vi "Main.vi"(8 "error in (no error)":errorcluster, 11 "TomoBase in":refnum<class "Tomo.lvclass">) -> (0 "error out":errorcluster, 3 "component":refnum<class "Tomo.lvclass">)   [LabVIEW 2012, in "Tomo.lvclass"]
doc: "Main VI of the component."
uses:
  Tomo.lvclass
  <vilib>/Distrio/Murmex/Murmex/command_enum.ctl
  Tomo.lvclass/Tomo.ctl
  <vilib>/Distrio/Murmex/InitialiseMessage/InitialiseMessage.lvclass
  <vilib>/Distrio/Murmex/TerminateMessage/TerminateMessage.lvclass
  <vilib>/Distrio/Murmex/ConfigureMessage/ConfigureMessage.lvclass
  <vilib>/Distrio/Murmex/Murmex/update_cluster.ctl
  <vilib>/Distrio/Murmex/StopMessage/StopMessage.lvclass
  <vilib>/Distrio/Murmex/GenericMessage/GenericMessage.lvclass
  <vilib>/Distrio/Murmex/Murmex/Set configure at initialise.vi
  <vilib>/Distrio/Murmex/Murmex/Set log reference.vi
  <vilib>/Distrio/Murmex/Murmex/Set VI reference.vi
  <vilib>/Distrio/Murmex/Murmex/Set write log to disk.vi
  <vilib>/Distrio/Murmex/Message/Add or replace parameter.vi
  <vilib>/Distrio/Murmex/Murmex/Murmex.lvclass
  <vilib>/Distrio/Murmex/Message/Message.lvclass
panel:
  in  "Tab Control":T1(tab)
  out "TB":dbl format="%#_2g"
  out "Tomography progress":dbl(slide) scale=0.0..1.0
  in  "experiment name":string
  in  "Volume map":T2(ring)
  in  "Z step size":dbl[unit]=1e-06
  in  "X step size":dbl[unit]=0.0005
  in  "Y step size":dbl[unit]=0.0005
  in  "# of views":dbl=1.0
  in  "starting angle":dbl[unit]
  in  "button::start":bool
  out "Estimated remaining time":dbl format="- %<%H:%M:%S>t"
  in  "Default focus":dbl[unit]
  in  "Pivotal X":dbl[unit]
  in  "Reverse stacks?":bool
  in  "X min":dbl[unit]
  in  "X max":dbl[unit]
  in  "Y min":dbl[unit]
  in  "Y max":dbl[unit]
  in  "Z min":dbl[unit]
  in  "Z max":dbl[unit]
  in  "Pre tomo volume file":path
  in  "Pre tomo binary images path":path
  in  "button::pretomo calc":bool
  in  "Custom volume path":path
  in  "Experimenter email address":string
  in  "Experimenter name":string
  in  "generic command":string
  in  "button::send command":bool
  out "log":string
  in  "ID":string="tomo"
  in  "command":T3
  in  "recipient":string
  in  "button::configure":bool
  in  "button::quit":bool
  in  "terminate?":bool
  # "Tomo\n\nImplemented by:\nLudovico Silvestri\nUniversity of Florence, Italy"
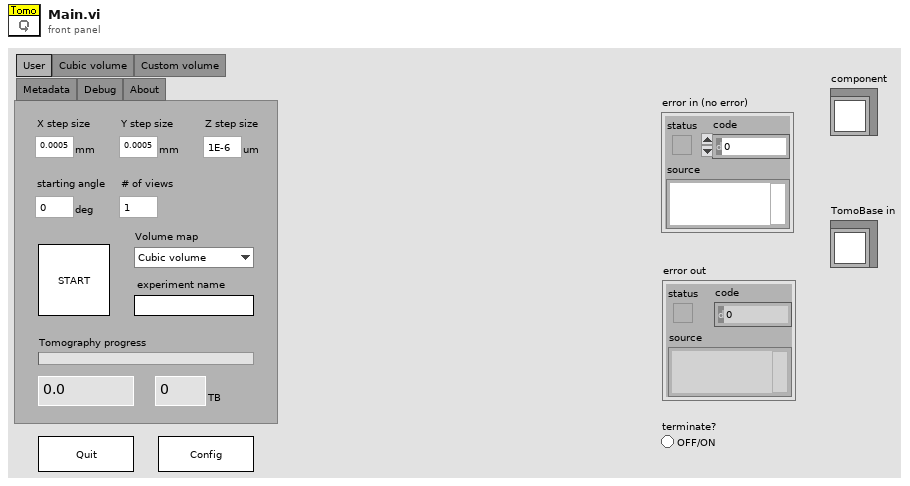
[diagram p1: front panel]
types:
  T1 = enum32{"User", "Cubic volume", "Custom volume", "Metadata", "Debug", "About"}
  T2 = enum16{"Cubic volume", "Custom volume", "Self-generate volume"}
  T3 = typedef "Murmex.lvlib/Murmex.lvclass/command_enum.ctl" = enum16{"null", "initialise", "reset", "terminate", "acknowledge", "update", "inspect", "inform", "proceed", "start", "stop", "fetch", "configure", "generic"}
  T4 = typedef "Murmex.lvlib/Murmex.lvclass/update_cluster.ctl" = cluster{"target ID":string, "key chains":string[], "values":variant[]}
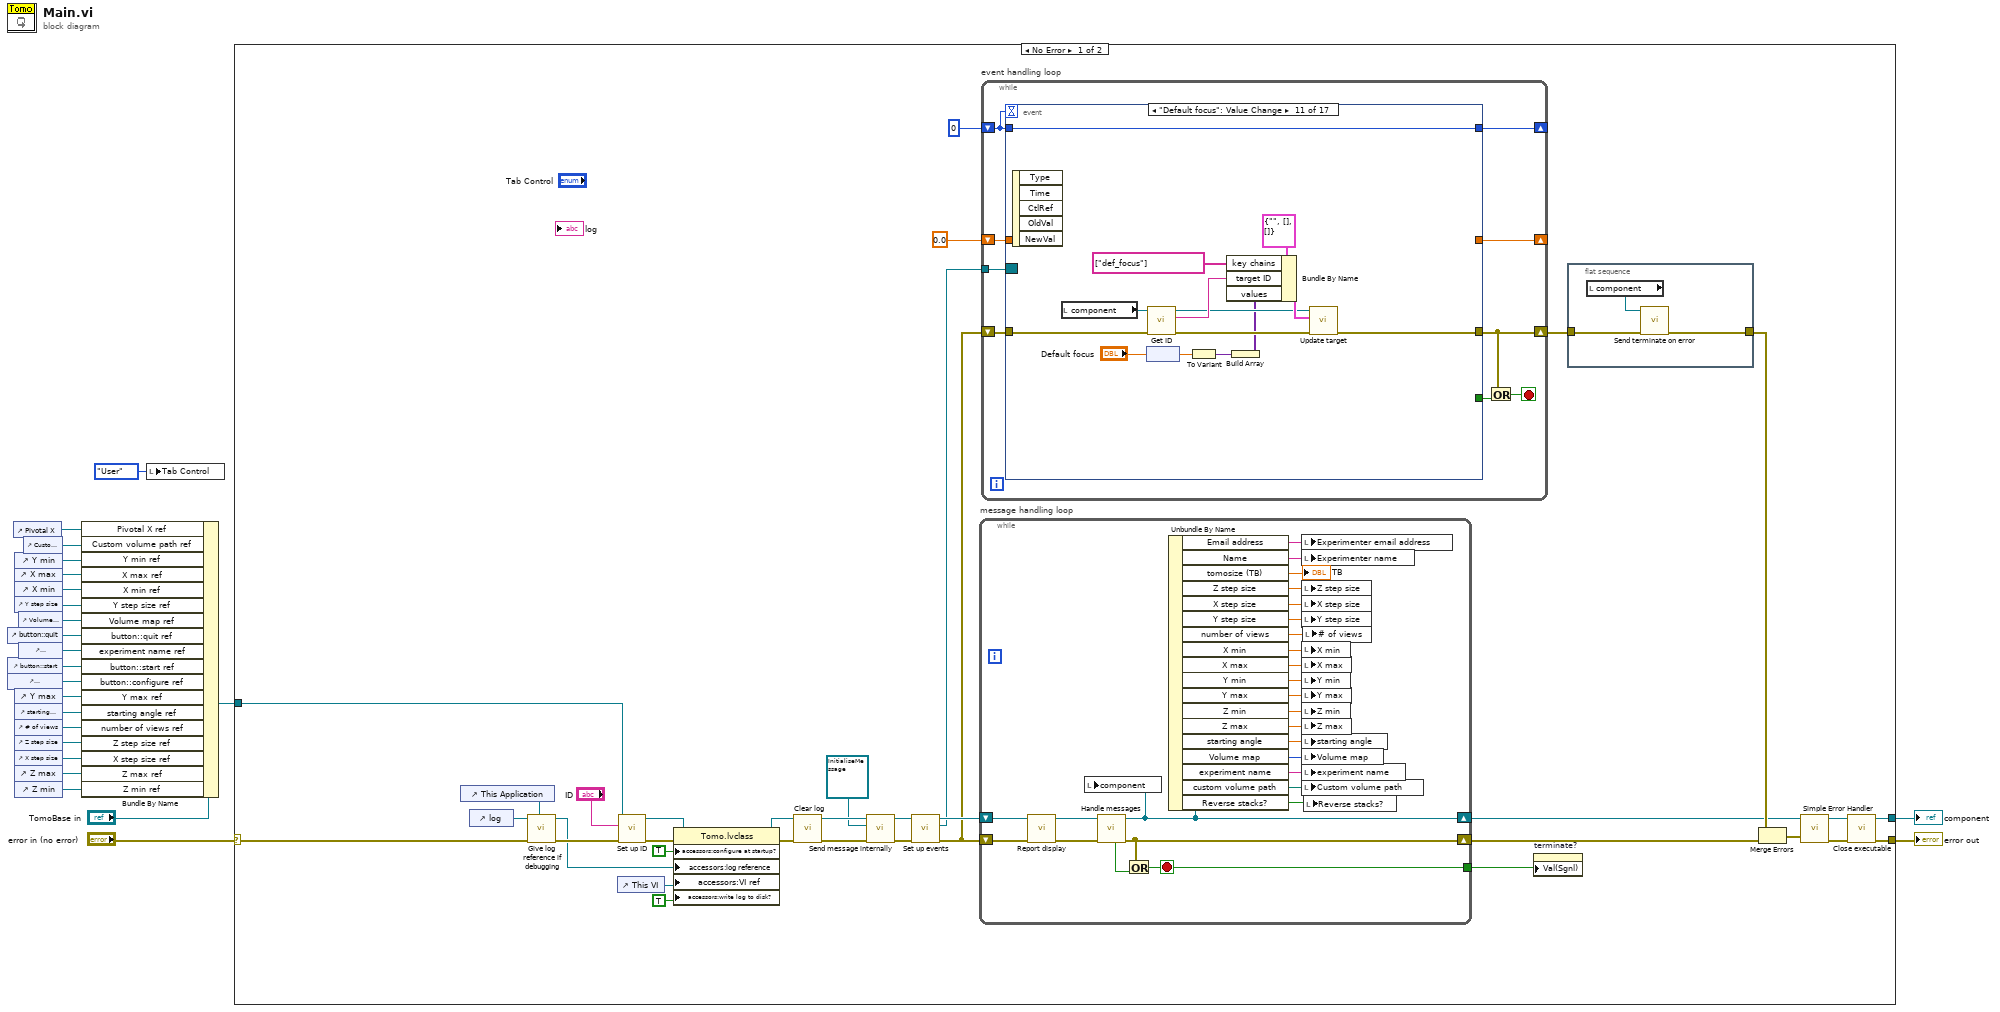
[diagram p0: block diagram]
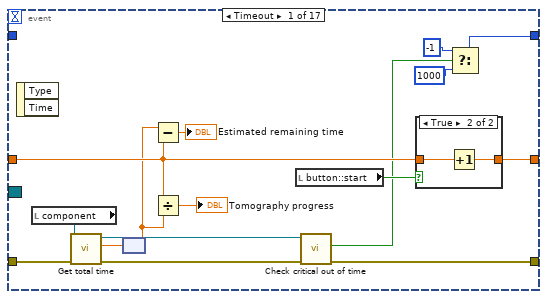
[diagram p2: hidden frame]
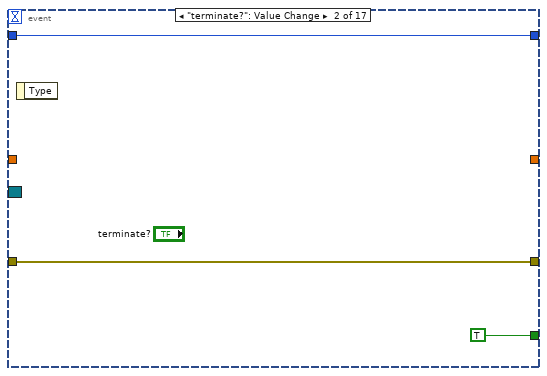
[diagram p4: hidden frame]
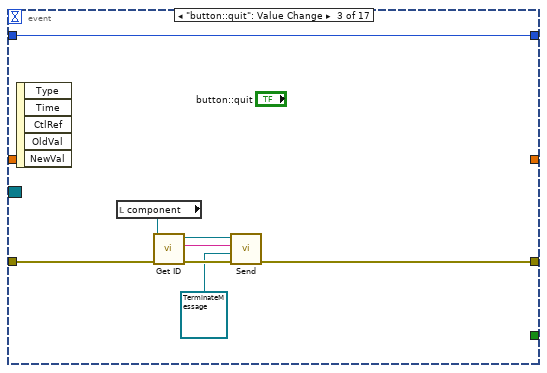
[diagram p5: hidden frame]
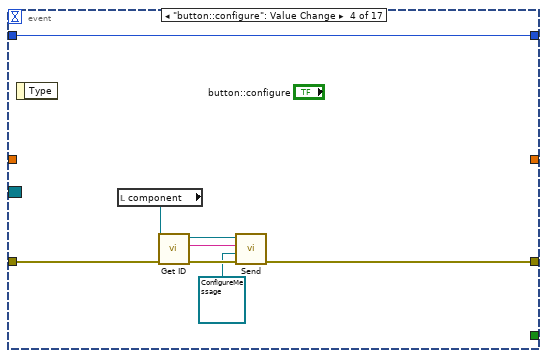
[diagram p6: hidden frame]
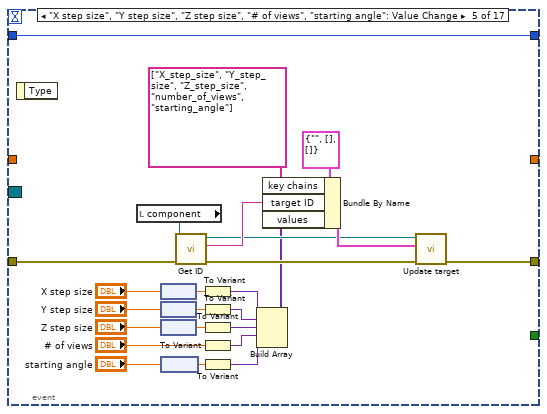
[diagram p7: hidden frame]
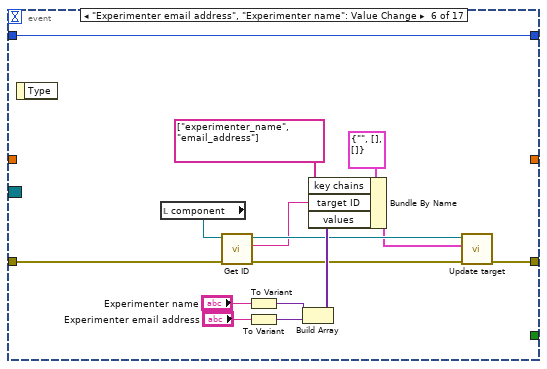
[diagram p8: hidden frame]
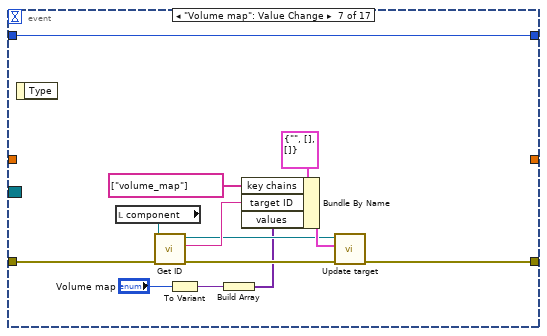
[diagram p9: hidden frame]
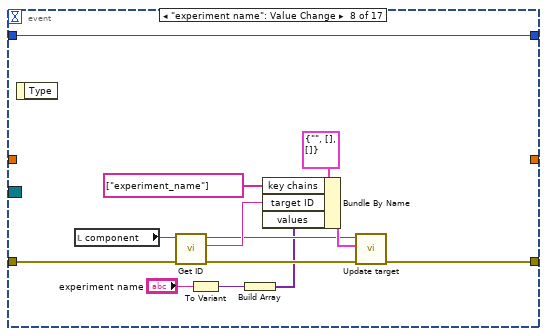
[diagram p10: hidden frame]
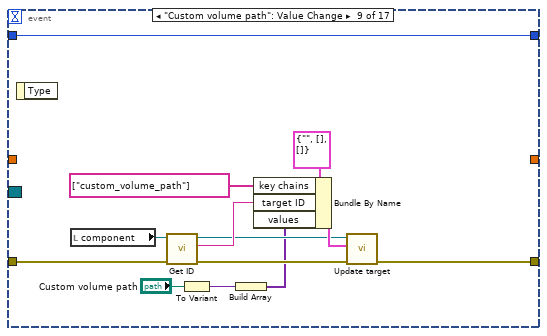
[diagram p11: hidden frame]
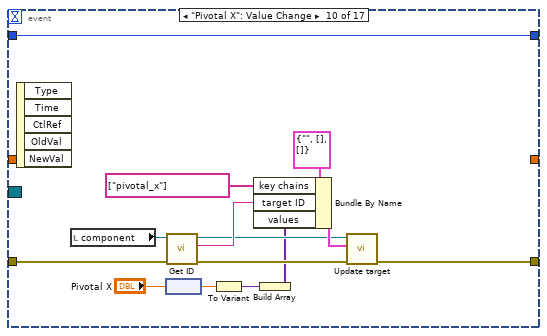
[diagram p12: hidden frame]
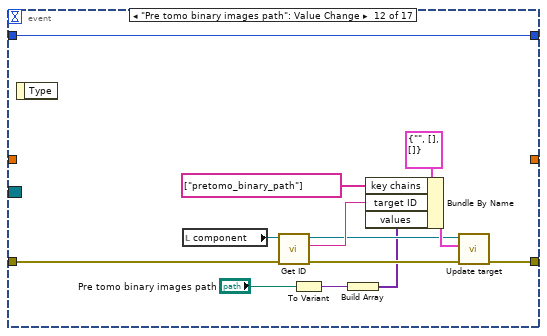
[diagram p13: hidden frame]
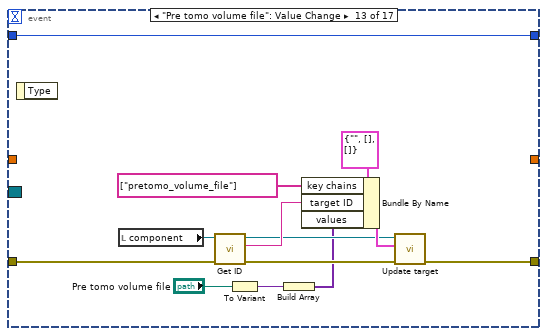
[diagram p14: hidden frame]
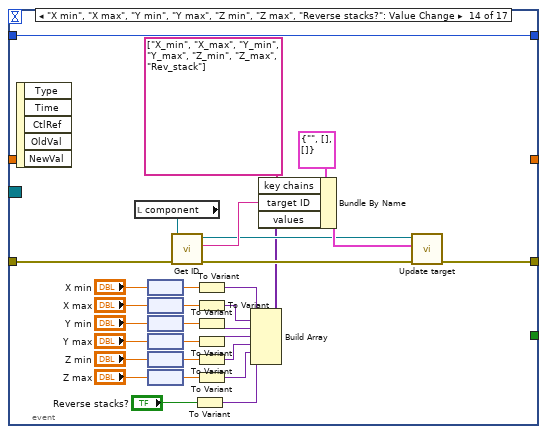
[diagram p15: hidden frame]
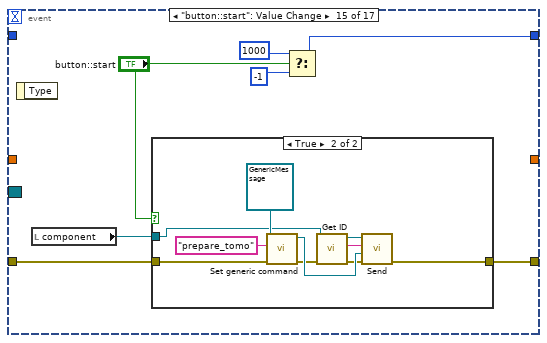
[diagram p16: hidden frame]
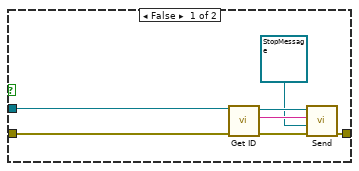
[diagram p17: hidden frame]
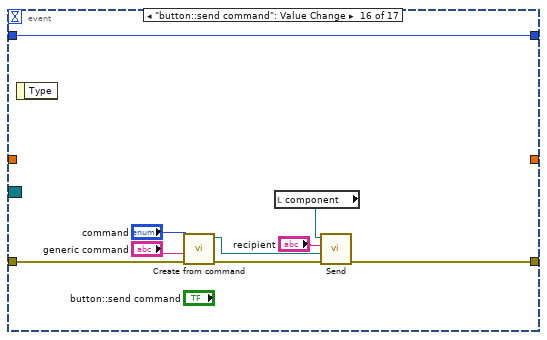
[diagram p18: hidden frame]
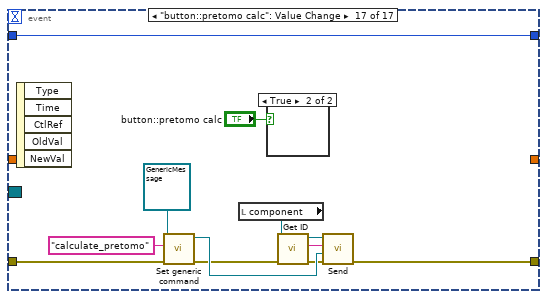
[diagram p19: hidden frame]
diagram:
  n1 = control-ref of="button::quit"() -> (w13:refnum<vi>)
  n2 = control-ref of="button::start"() -> (w11:refnum<vi>)
  n3 = control-ref of="button::configure"() -> (w10:refnum<vi>)
  n4 = control-ref of="Pivotal X"() -> (w1:refnum<vi>)
  n5 = control-ref of="Y min"() -> (w18:refnum<vi>)
  n6 = control-ref of="X max"() -> (w17:refnum<vi>)
  n7 = control-ref of="X min"() -> (w16:refnum<vi>)
  n8 = control-ref of="Y step size"() -> (w15:refnum<vi>)
  n9 = control-ref of="Y max"() -> (w9:refnum<vi>)
  n10 = control-ref of="starting angle"() -> (w8:refnum<vi>)
  n11 = control-ref of="# of views"() -> (w7:refnum<vi>)
  n12 = control-ref of="Z step size"() -> (w6:refnum<vi>)
  n13 = control-ref of="X step size"() -> (w5:refnum<vi>)
  n14 = control-ref of="Z max"() -> (w4:refnum<vi>)
  n15 = control-ref of="Z min"() -> (w3:refnum<vi>)
  n16 = control-ref of="Volume map"() -> (w14:refnum<vi>)
  n17 = control-ref of="experiment name"() -> (w12:refnum<vi>)
  n18 = control-ref of="Custom volume path"() -> (w19:refnum<vi>)
  n19 = Bundle By Name(cluster="TomoBase in", "Pivotal X ref"=w1, "Custom volume path ref"=w19, "Y min ref"=w18, "X max ref"=w17, "X min ref"=w16, "Y step size ref"=w15, "Volume map ref"=w14, "button::quit ref"=w13, "experiment name ref"=w12, "button::start ref"=w11, "button::configure ref"=w10, "Y max ref"=w9, "starting angle ref"=w8, "number of views ref"=w7, "Z step size ref"=w6, "X step size ref"=w5, "Z max ref"=w4, "Z min ref"=w3) -> (w20:refnum<class "Tomo.lvclass">)
  n20 = local write "Tab Control"(T1."User" ("Tab Control")) -> ()
  n21 = case shown="No Error" "error in (no error)" {
    selector: "error in (no error)" -> [w29 w343]
    tunnel: w20 -> [w54 w342]
    tunnel: [w34 w343] -> w23
    tunnel: [w32 w342] -> w22
    frame No Error {
      n22 = control-ref of="This Application"() -> (w26:refnum<vi>)
      n23 = control-ref of="log"() -> (w28:refnum<vi>)
      n24 = call "Give log reference if debugging.vi"("application ref"=w26, "error in (no error)"=w29, "log reference in"=w28) -> ("error out"=w30:errorcluster, "log reference out"=w27:refnum<vi>)  [unwired: 6 in, 1 out]
      n25 = control-ref of="This VI"() -> (w56:refnum<vi>)
      n26 = call <vilib>:"Set up ID.vi"("error in (no error)"=w30, "component ID"="ID", "MurmexBase in"=w54) -> ("error out"=w55:errorcluster, "MurmexBase out"=w52:refnum<class "Tomo.lvclass">)  [unwired: 6 in, 1 out]
      n27 = property class="Tomo.lvclass"(reference=w52, error in=w55, "accessors:configure at startup?"=TRUE ("configure at startup?"), "accessors:log reference"=w27, "accessors:VI ref"=w56, "accessors:write log to disk?"=TRUE ("write log to disk?")) -> (reference out=w50:refnum<class "Tomo.lvclass">, error out=w51:errorcluster)
      n28 = call <vilib>:"Clear log.vi"("error in (no error)"=w51, "MurmexBase in"=w50) -> ("error out"=w49:errorcluster, "MurmexBase out"=w48:refnum<class "Tomo.lvclass">)  [unwired: 8 in]
      n29 = call <vilib>:"Send message internally.vi"("error in (no error)"=w49, "Message"=refnum<class "InitialiseMessage.lvclass"> refnum ("Message in"), "Murmex in"=w48) -> ("error out"=w46:errorcluster, "Murmex out"=w45:refnum<class "Tomo.lvclass">)  [unwired: 7 in]
      n30 = call <vilib>:"Set up events.vi"("error in (no error)"=w46, "MurmexBase in"=w45) -> ("error out"=w43:errorcluster, "Event Registration Refnum"=w42:refnum<event-registration>, "MurmexBase out"=w44:refnum<class "Tomo.lvclass">)  [unwired: 7 in]
      n31 = while "message handling loop" {
        shift-right: [w322] -> w39
        shift-left: w43 -> [w320]
        shift-right: [w321] -> w33
        shift-left: w44 -> [w318]
        tunnel: [w340] -> w35
        stop <- w340 stop-if-true
        n32 = call-dynamic "Report display.vi"("error in (no error)"=w320, "Tomo in"=w318) -> ("error out"=w319:errorcluster, "Tomo out"=w317:refnum<class "Tomo.lvclass">)  [unwired: 8 in]
        n33 = call <vilib>:"Handle messages.vi"("error in (no error)"=w319, "Murmex in"=w317) -> ("error out"=w322:errorcluster, "Murmex out"=w321:refnum<class "Tomo.lvclass">, "terminated?"=w341:bool)  [unwired: 7 in]
        n34 = local write "component"(w321) -> ()
        n35 = Or(x=w322, y=w341) -> (x .or. y?=w340:bool)
        n36 = Unbundle By Name(w321) -> ("Email address"=w323:string, "Name"=w324:string, "tomosize (TB)"=→"TB":dbl, "Z step size"=w331:dbl[unit], "X step size"=w333:dbl[unit], "Y step size"=w332:dbl[unit], "number of views"=w330:dbl, "X min"=w339:dbl[unit], "X max"=w338:dbl[unit], "Y min"=w337:dbl[unit], "Y max"=w336:dbl[unit], "Z min"=w335:dbl[unit], "Z max"=w334:dbl[unit], "starting angle"=w329:dbl[unit], "Volume map"=w328:T2, "experiment name"=w327:string, "custom volume path"=w326:path, "Reverse stacks?"=w316:bool)
        n37 = local write "Experimenter email address"(w323) -> ()
        n38 = local write "Experimenter name"(w324) -> ()
        n39 = local write "Z step size"(w331) -> ()
        n40 = local write "X step size"(w333) -> ()
        n41 = local write "Y step size"(w332) -> ()
        n42 = local write "X min"(w339) -> ()
        n43 = local write "X max"(w338) -> ()
        n44 = local write "Y min"(w337) -> ()
        n45 = local write "Y max"(w336) -> ()
        n46 = local write "Z min"(w335) -> ()
        n47 = local write "Z max"(w334) -> ()
        n48 = local write "starting angle"(w329) -> ()
        n49 = local write "Volume map"(w328) -> ()
        n50 = local write "experiment name"(w327) -> ()
        n51 = local write "Custom volume path"(w326) -> ()
        n52 = local write "# of views"(w330) -> ()
        n53 = local write "Reverse stacks?"(w316) -> ()
      }
      n54 = while "event handling loop" {
        shift-right: [w64] -> w40
        shift-left: w43 -> [w69]
        tunnel: w42 -> [w68]
        shift-right: [w66] -> _
        shift-left: 0 -> [w67]
        shift-right: [w61] -> _
        shift-left: 0.0 -> [w62]
        stop <- w63 stop-if-true
        n55 = event shown="[10] \"Default focus\": Value Change" {
          selector: w68 -> [_ _ _ _ _ _ _ _ _ _ _ _ _ _ _ _ _]
          dyn-events: _ -> [_ _ _ _ _ _ _ _ _ _ _ _ _ _ _ _ _]
          timeout: w67 -> [_ _ _ _ _ _ _ _ _ _ _ _ _ _ _ _ _]
          tunnel: [w75 w89 w96 w102 w130 w138 w154 w162 w178 w192 w206 w219 w232 w265 w277 w296 w306] -> w64
          tunnel: w69 -> [w85 w89 w98 w103 w128 w137 w156 w165 w177 w191 w205 w218 w231 w263 w276 w302 w307]
          tunnel: w67 -> [_ w88 w91 w99 w111 w132 w153 w161 w173 w188 w202 w215 w228 w249 _ w295 w304]
          tunnel: [w70 w88 w91 w99 w111 w132 w153 w161 w173 w188 w202 w215 w228 w249 w271 w295 w304] -> w66
          tunnel: [_ TRUE _ _ _ _ _ _ _ _ _ _ _ _ _ _ _] -> w65
          tunnel: w62 -> [w83 _ _ _ _ _ _ _ _ _ _ _ _ _ _ _ _]
          tunnel: [w82 _ _ _ _ _ _ _ _ _ _ _ _ _ _ _ _] -> w61
          event Timeout {
            n56 = event-data() -> ()  [unwired: 1 in, 2 out]
            n57 = local read "component"() -> (w81:refnum<class "Tomo.lvclass">)
            n58 = call-dynamic "Get total time.vi"("error in (no error)"=w85, "Tomo in"=w81) -> ("error out"=w84:errorcluster, "Total time"=w80:dbl[unit], "Tomo out"=w74:refnum<class "Tomo.lvclass">)  [unwired: 7 in]
            n59 = node(w80) -> (w78:dbl)
            n60 = Subtract(x=w78, y=w83) -> (x-y=→"Estimated remaining time":dbl)
            n61 = Divide(x=w83, y=w78) -> (x/y=→"Tomography progress":dbl)
            n62 = local read "button::start"() -> (w76:bool)
            n63 = call-dynamic "Check critical out of time.vi"("error in (no error)"=w84, "Tomo in"=w74) -> ("error out"=w75:errorcluster, "critical issue?"=w73:bool)  [unwired: 7 in, 1 out]
            n64 = case shown="True" w76 {
              tunnel: w83 -> [_ w87]
              tunnel: [_ w86] -> w82
              frame False {
              }
              frame True {
                n65 = Increment(x=w87) -> (x+1=w86:dbl)
              }
            }
            n66 = Select(t=-1, s=w73, f=1000) -> (s? t:f=w70:i32)
          }
          event "terminate?": Value Change {
            n67 = event-data() -> ()  [unwired: 1 in, 1 out]
          }
          event "button::quit": Value Change {
            n68 = event-data() -> ()  [unwired: 1 in, 5 out]
            n69 = local read "component"() -> (w95:refnum<class "Tomo.lvclass">)
            n70 = call <vilib>:"Get ID.vi"("error in (no error)"=w98, "Murmex in"=w95) -> ("error out"=w97:errorcluster, "component id"=w93:string, "Murmex out"=w94:refnum<class "Tomo.lvclass">)  [unwired: 7 in]
            n71 = call <vilib>:"Send.vi"("error in (no error)"=w97, "Message"=refnum<class "TerminateMessage.lvclass"> refnum ("Distrio Murmex 1.1:TerminateMessage"), "recipient"=w93, "Murmex in"=w94) -> ("error out"=w96:errorcluster)  [unwired: 6 in, 1 out]
          }
          event "button::configure": Value Change {
            n72 = event-data() -> ()  [unwired: 1 in, 1 out]
            n73 = local read "component"() -> (w101:refnum<class "Tomo.lvclass">)
            n74 = call <vilib>:"Get ID.vi"("error in (no error)"=w103, "Murmex in"=w101) -> ("error out"=w106:errorcluster, "component id"=w104:string, "Murmex out"=w105:refnum<class "Tomo.lvclass">)  [unwired: 7 in]
            n75 = call <vilib>:"Send.vi"("error in (no error)"=w106, "Message"=refnum<class "ConfigureMessage.lvclass"> refnum ("Distrio Murmex 1.1:ConfigureMessage"), "recipient"=w104, "Murmex in"=w105) -> ("error out"=w102:errorcluster)  [unwired: 6 in, 1 out]
          }
          event "X step size", "Y step size", "Z step size", "# of views", "starting angle": Value Change {
            n76 = event-data() -> ()  [unwired: 1 in, 1 out]
            n77 = local read "component"() -> (w126:refnum<class "Tomo.lvclass">)
            n78 = node("X step size") -> (w110:dbl)
            n79 = node("Y step size") -> (w109:dbl)
            n80 = node("Z step size") -> (w108:dbl)
            n81 = node("starting angle") -> (w107:dbl)
            n82 = call <vilib>:"Get ID.vi"("error in (no error)"=w128, "Murmex in"=w126) -> ("error out"=w129:errorcluster, "component id"=w127:string, "Murmex out"=w124:refnum<class "Tomo.lvclass">)  [unwired: 7 in]
            n83 = To Variant(anything=w110) -> (Variant=w114:variant)
            n84 = To Variant(anything=w109) -> (Variant=w115:variant)
            n85 = To Variant(anything=w108) -> (Variant=w118:variant)
            n86 = To Variant(anything="# of views") -> (Variant=w117:variant)
            n87 = To Variant(anything=w107) -> (Variant=w116:variant)
            n88 = Build Array(w114, w115, w118, w117, w116) -> (w113:variant[])
            n89 = Bundle By Name(cluster=T4 {"target ID"="", "key chains"=[], "values"=[]} ("update cluster"), "key chains"=string[] ["X_step_size", "Y_step_size", "Z_step_size", "number_of_views", "starting_angle"], "target ID"=w127, "values"=w113) -> (w125:T4)
            n90 = call <vilib>:"Update target.vi"("error in (no error)"=w129, "update cluster"=w125, "MurmexBase in"=w124) -> ("error out"=w130:errorcluster)  [unwired: 7 in, 1 out]
          }
          event "Experimenter email address", "Experimenter name": Value Change {
            n91 = event-data() -> ()  [unwired: 1 in, 1 out]
            n92 = local read "component"() -> (w133:refnum<class "Tomo.lvclass">)
            n93 = call <vilib>:"Get ID.vi"("error in (no error)"=w137, "Murmex in"=w133) -> ("error out"=w140:errorcluster, "component id"=w141:string, "Murmex out"=w143:refnum<class "Tomo.lvclass">)  [unwired: 7 in]
            n94 = To Variant(anything="Experimenter name") -> (Variant=w145:variant)
            n95 = To Variant(anything="Experimenter email address") -> (Variant=w144:variant)
            n96 = Build Array(w145, w144) -> (w146:variant[])
            n97 = Bundle By Name(cluster=T4 {"target ID"="", "key chains"=[], "values"=[]} ("update cluster"), "key chains"=string[] ["experimenter_name", "email_address"], "target ID"=w141, "values"=w146) -> (w142:T4)
            n98 = call <vilib>:"Update target.vi"("error in (no error)"=w140, "update cluster"=w142, "MurmexBase in"=w143) -> ("error out"=w138:errorcluster)  [unwired: 7 in, 1 out]
          }
          event "Volume map": Value Change {
            n99 = event-data() -> ()  [unwired: 1 in, 1 out]
            n100 = local read "component"() -> (w147:refnum<class "Tomo.lvclass">)
            n101 = call <vilib>:"Get ID.vi"("error in (no error)"=w156, "Murmex in"=w147) -> ("error out"=w155:errorcluster, "component id"=w159:string, "Murmex out"=w157:refnum<class "Tomo.lvclass">)  [unwired: 7 in]
            n102 = To Variant(anything="Volume map") -> (Variant=w152:variant)
            n103 = Build Array(w152) -> (w151:variant[])
            n104 = Bundle By Name(cluster=T4 {"target ID"="", "key chains"=[], "values"=[]} ("update cluster"), "key chains"=string[] ["volume_map"], "target ID"=w159, "values"=w151) -> (w158:T4)
            n105 = call <vilib>:"Update target.vi"("error in (no error)"=w155, "update cluster"=w158, "MurmexBase in"=w157) -> ("error out"=w154:errorcluster)  [unwired: 7 in, 1 out]
          }
          event "experiment name": Value Change {
            n106 = event-data() -> ()  [unwired: 1 in, 1 out]
            n107 = local read "component"() -> (w160:refnum<class "Tomo.lvclass">)
            n108 = call <vilib>:"Get ID.vi"("error in (no error)"=w165, "Murmex in"=w160) -> ("error out"=w169:errorcluster, "component id"=w172:string, "Murmex out"=w170:refnum<class "Tomo.lvclass">)  [unwired: 7 in]
            n109 = To Variant(anything="experiment name") -> (Variant=w168:variant)
            n110 = Build Array(w168) -> (w167:variant[])
            n111 = Bundle By Name(cluster=T4 {"target ID"="", "key chains"=[], "values"=[]} ("update cluster"), "key chains"=string[] ["experiment_name"], "target ID"=w172, "values"=w167) -> (w171:T4)
            n112 = call <vilib>:"Update target.vi"("error in (no error)"=w169, "update cluster"=w171, "MurmexBase in"=w170) -> ("error out"=w162:errorcluster)  [unwired: 7 in, 1 out]
          }
          event "Custom volume path": Value Change {
            n113 = event-data() -> ()  [unwired: 1 in, 1 out]
            n114 = local read "component"() -> (w175:refnum<class "Tomo.lvclass">)
            n115 = call <vilib>:"Get ID.vi"("error in (no error)"=w177, "Murmex in"=w175) -> ("error out"=w182:errorcluster, "component id"=w185:string, "Murmex out"=w183:refnum<class "Tomo.lvclass">)  [unwired: 7 in]
            n116 = To Variant(anything="Custom volume path") -> (Variant=w181:variant)
            n117 = Build Array(w181) -> (w180:variant[])
            n118 = Bundle By Name(cluster=T4 {"target ID"="", "key chains"=[], "values"=[]} ("update cluster"), "key chains"=string[] ["custom_volume_path"], "target ID"=w185, "values"=w180) -> (w184:T4)
            n119 = call <vilib>:"Update target.vi"("error in (no error)"=w182, "update cluster"=w184, "MurmexBase in"=w183) -> ("error out"=w178:errorcluster)  [unwired: 7 in, 1 out]
          }
          event "Pivotal X": Value Change {
            n120 = event-data() -> ()  [unwired: 1 in, 5 out]
            n121 = local read "component"() -> (w190:refnum<class "Tomo.lvclass">)
            n122 = node("Pivotal X") -> (w186:dbl)
            n123 = call <vilib>:"Get ID.vi"("error in (no error)"=w191, "Murmex in"=w190) -> ("error out"=w196:errorcluster, "component id"=w199:string, "Murmex out"=w197:refnum<class "Tomo.lvclass">)  [unwired: 7 in]
            n124 = To Variant(anything=w186) -> (Variant=w195:variant)
            n125 = Build Array(w195) -> (w194:variant[])
            n126 = Bundle By Name(cluster=T4 {"target ID"="", "key chains"=[], "values"=[]} ("update cluster"), "key chains"=string[] ["pivotal_x"], "target ID"=w199, "values"=w194) -> (w198:T4)
            n127 = call <vilib>:"Update target.vi"("error in (no error)"=w196, "update cluster"=w198, "MurmexBase in"=w197) -> ("error out"=w192:errorcluster)  [unwired: 7 in, 1 out]
          }
          event "Default focus": Value Change {
            n128 = event-data() -> ()  [unwired: 1 in, 5 out]
            n129 = local read "component"() -> (w204:refnum<class "Tomo.lvclass">)
            n130 = node("Default focus") -> (w201:dbl)
            n131 = call <vilib>:"Get ID.vi"("error in (no error)"=w205, "Murmex in"=w204) -> ("error out"=w210:errorcluster, "component id"=w213:string, "Murmex out"=w211:refnum<class "Tomo.lvclass">)  [unwired: 7 in]
            n132 = To Variant(anything=w201) -> (Variant=w209:variant)
            n133 = Build Array(w209) -> (w208:variant[])
            n134 = Bundle By Name(cluster=T4 {"target ID"="", "key chains"=[], "values"=[]} ("update cluster"), "key chains"=string[] ["def_focus"], "target ID"=w213, "values"=w208) -> (w212:T4)
            n135 = call <vilib>:"Update target.vi"("error in (no error)"=w210, "update cluster"=w212, "MurmexBase in"=w211) -> ("error out"=w206:errorcluster)  [unwired: 7 in, 1 out]
          }
          event "Pre tomo binary images path": Value Change {
            n136 = event-data() -> ()  [unwired: 1 in, 1 out]
            n137 = local read "component"() -> (w217:refnum<class "Tomo.lvclass">)
            n138 = call <vilib>:"Get ID.vi"("error in (no error)"=w218, "Murmex in"=w217) -> ("error out"=w223:errorcluster, "component id"=w226:string, "Murmex out"=w224:refnum<class "Tomo.lvclass">)  [unwired: 7 in]
            n139 = To Variant(anything="Pre tomo binary images path") -> (Variant=w222:variant)
            n140 = Build Array(w222) -> (w221:variant[])
            n141 = Bundle By Name(cluster=T4 {"target ID"="", "key chains"=[], "values"=[]} ("update cluster"), "key chains"=string[] ["pretomo_binary_path"], "target ID"=w226, "values"=w221) -> (w225:T4)
            n142 = call <vilib>:"Update target.vi"("error in (no error)"=w223, "update cluster"=w225, "MurmexBase in"=w224) -> ("error out"=w219:errorcluster)  [unwired: 7 in, 1 out]
          }
          event "Pre tomo volume file": Value Change {
            n143 = event-data() -> ()  [unwired: 1 in, 1 out]
            n144 = local read "component"() -> (w230:refnum<class "Tomo.lvclass">)
            n145 = call <vilib>:"Get ID.vi"("error in (no error)"=w231, "Murmex in"=w230) -> ("error out"=w236:errorcluster, "component id"=w239:string, "Murmex out"=w237:refnum<class "Tomo.lvclass">)  [unwired: 7 in]
            n146 = To Variant(anything="Pre tomo volume file") -> (Variant=w235:variant)
            n147 = Build Array(w235) -> (w234:variant[])
            n148 = Bundle By Name(cluster=T4 {"target ID"="", "key chains"=[], "values"=[]} ("update cluster"), "key chains"=string[] ["pretomo_volume_file"], "target ID"=w239, "values"=w234) -> (w238:T4)
            n149 = call <vilib>:"Update target.vi"("error in (no error)"=w236, "update cluster"=w238, "MurmexBase in"=w237) -> ("error out"=w232:errorcluster)  [unwired: 7 in, 1 out]
          }
          event "X min", "X max", "Y min", "Y max", "Z min", "Z max", "Reverse stacks?": Value Change {
            n150 = event-data() -> ()  [unwired: 1 in, 5 out]
            n151 = local read "component"() -> (w262:refnum<class "Tomo.lvclass">)
            n152 = node("X min") -> (w248:dbl)
            n153 = node("X max") -> (w247:dbl)
            n154 = node("Y min") -> (w246:dbl)
            n155 = node("Y max") -> (w245:dbl)
            n156 = node("Z min") -> (w243:dbl)
            n157 = node("Z max") -> (w242:dbl)
            n158 = call <vilib>:"Get ID.vi"("error in (no error)"=w263, "Murmex in"=w262) -> ("error out"=w264:errorcluster, "component id"=w269:string, "Murmex out"=w267:refnum<class "Tomo.lvclass">)  [unwired: 7 in]
            n159 = To Variant(anything="Reverse stacks?") -> (Variant=w240:variant)
            n160 = To Variant(anything=w248) -> (Variant=w258:variant)
            n161 = To Variant(anything=w247) -> (Variant=w259:variant)
            n162 = To Variant(anything=w246) -> (Variant=w261:variant)
            n163 = To Variant(anything=w245) -> (Variant=w260:variant)
            n164 = To Variant(anything=w243) -> (Variant=w251:variant)
            n165 = To Variant(anything=w242) -> (Variant=w250:variant)
            n166 = Build Array(w258, w259, w261, w260, w251, w250, w240) -> (w257:variant[])
            n167 = Bundle By Name(cluster=T4 {"target ID"="", "key chains"=[], "values"=[]} ("update cluster"), "key chains"=string[] ["X_min", "X_max", "Y_min", "Y_max", "Z_min", "Z_max", "Rev_stack"], "target ID"=w269, "values"=w257) -> (w268:T4)
            n168 = call <vilib>:"Update target.vi"("error in (no error)"=w264, "update cluster"=w268, "MurmexBase in"=w267) -> ("error out"=w265:errorcluster)  [unwired: 7 in, 1 out]
          }
          event "button::start": Value Change {
            n169 = event-data() -> ()  [unwired: 1 in, 1 out]
            n170 = local read "component"() -> (w275:refnum<class "Tomo.lvclass">)
            n171 = case shown="True" "button::start" {
              tunnel: [w282 w285] -> w277
              tunnel: w276 -> [w280 w287]
              tunnel: w275 -> [w278 w286]
              frame False {
                n172 = call <vilib>:"Get ID.vi"("error in (no error)"=w280, "Murmex in"=w278) -> ("error out"=w281:errorcluster, "component id"=w283:string, "Murmex out"=w284:refnum<class "Tomo.lvclass">)  [unwired: 7 in]
                n173 = call <vilib>:"Send.vi"("error in (no error)"=w281, "Message"=refnum<class "StopMessage.lvclass"> refnum ("Distrio Murmex 1.1:StopMessage"), "recipient"=w283, "Murmex in"=w284) -> ("error out"=w282:errorcluster)  [unwired: 6 in, 1 out]
              }
              frame True {
                n174 = call <vilib>:"Set generic command.vi"("error in (no error)"=w287, "generic command"="prepare_tomo", "GenericMessage in"=refnum<class "GenericMessage.lvclass"> refnum ("Message in")) -> ("error out"=w289:errorcluster, "GenericMessage out"=w293:refnum<class "GenericMessage.lvclass">)  [unwired: 7 in]
                n175 = call <vilib>:"Get ID.vi"("error in (no error)"=w289, "Murmex in"=w286) -> ("error out"=w290:errorcluster, "component id"=w292:string, "Murmex out"=w291:refnum<class "Tomo.lvclass">)  [unwired: 7 in]
                n176 = call <vilib>:"Send.vi"("error in (no error)"=w290, "Message"=w293, "recipient"=w292, "Murmex in"=w291) -> ("error out"=w285:errorcluster)  [unwired: 6 in, 1 out]
              }
            }
            n177 = Select(t=1000, s="button::start", f=-1) -> (s? t:f=w271:i32)
          }
          event "button::send command": Value Change {
            n178 = event-data() -> ()  [unwired: 1 in, 1 out]
            n179 = call <vilib>:"Create from command.vi"("error in (no error)"=w302, "generic command"="generic command", "command"="command") -> ("error out"=w297:errorcluster, "Message out"=w298:refnum<class "Message.lvclass">)  [unwired: 7 in]
            n180 = local read "component"() -> (w299:refnum<class "Tomo.lvclass">)
            n181 = call <vilib>:"Send.vi"("error in (no error)"=w297, "Message"=w298, "recipient"="recipient", "Murmex in"=w299) -> ("error out"=w296:errorcluster)  [unwired: 6 in, 1 out]
          }
          event "button::pretomo calc": Value Change {
            n182 = event-data() -> ()  [unwired: 1 in, 5 out]
            n183 = call <vilib>:"Set generic command.vi"("error in (no error)"=w307, "generic command"="calculate_pretomo", "GenericMessage in"=refnum<class "GenericMessage.lvclass"> refnum ("Message in")) -> ("error out"=w309:errorcluster, "GenericMessage out"=w313:refnum<class "GenericMessage.lvclass">)  [unwired: 7 in]
            n184 = local read "component"() -> (w305:refnum<class "Tomo.lvclass">)
            n185 = case shown="True" "button::pretomo calc" {
              frame False {
              }
              frame True {
              }
            }
            n186 = call <vilib>:"Get ID.vi"("error in (no error)"=w309, "Murmex in"=w305) -> ("error out"=w310:errorcluster, "component id"=w312:string, "Murmex out"=w311:refnum<class "Tomo.lvclass">)  [unwired: 7 in]
            n187 = call <vilib>:"Send.vi"("error in (no error)"=w310, "Message"=w313, "recipient"=w312, "Murmex in"=w311) -> ("error out"=w306:errorcluster)  [unwired: 6 in, 1 out]
          }
        }
        n188 = Or(x=w64, y=w65) -> (x .or. y?=w63:bool)
      }
      n189 = property on="terminate?" class="Bool (strict)"("Val(Sgnl)"=w35) -> ()  [unwired: 2 in, 2 out]
      n190 = flat-sequence {
        tunnel: w40 -> [w60]
        tunnel: [w58] -> w38
        frame #0 {
          n191 = local read "component"() -> (w59:refnum<class "Tomo.lvclass">)
          n192 = call <vilib>:"Send terminate on error.vi"("error in (no error)"=w60, "Murmex in"=w59) -> ("error out"=w58:errorcluster)  [unwired: 8 in, 1 out]
        }
      }
      n193 = Merge Errors(w38, w39) -> (w37:errorcluster)
      n194 = call <vilib>:"Simple Error Handler.vi"("error in (no error)"=w37) -> ("error out"=w36:errorcluster)  [unwired: 4 in, 4 out]
      n195 = call <vilib>:"Close executable.vi"("error in (no error)"=w36, "MurmexBase in"=w33) -> ("error out"=w34:errorcluster, "MurmexBase out"=w32:refnum<class "Tomo.lvclass">)  [unwired: 8 in]
    }
    frame Error {
    }
  }
  "error out" <- w23
  "component" <- w22
